vi "pclose serial.vi"(11 "resourceId":i32) -> (2 "nook":i32, 3 "resourceId out":i32)   [LabVIEW 2010, in "libcommon_serial.lvlib"]
doc: "close a previously open serial channel\n\nint pclose_serial(pserial_handle_t h);"
uses:
  <userlib>/libcommon_serial/libcommon_serial.lvlib
  <userlib>/libcommon_serial/libcommon_serial.so
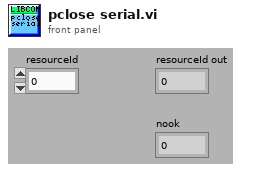
[diagram p1: front panel]
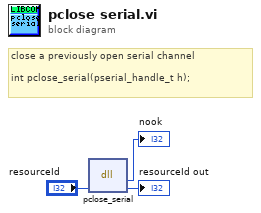
[diagram p0: block diagram]
diagram:
  # "close a previously open serial channel\n\nint pclose_serial(pserial_handle_t h);"
  n1 = dll-call lib="usr/local/natinst/LabVIEW-2010/user.lib/libcommon_serial/libcommon_serial.*" fn="pclose_serial"("resourceId"="resourceId") -> (→"nook":i32, "resourceId"=→"resourceId out":i32)  [unwired: 3 in, 2 out]
